vi "Dashboard Main.vi"() -> ()   [LabVIEW 2017]
uses:
  <vilib>/Utility/miscctls.llb/LVRowAndColumnTypeDef.ctl
  <vilib>/event_ctls.llb/eventvkey.ctl
  <vilib>/Rock Robotics/Network Tables/NT Read Numeric Array.vi
  <vilib>/Rock Robotics/WPI/Dashboard/WPI_DashboardLogging Global.vi
panel:
  in  "Camera Settings Right":T1={"Frame Rate"=30, "Compression"=30, "Size"=1, "DB Camera Config"=FALSE} {"Frame Rate" scale=1.0..30.0; "Compression" scale=100.0..-1.0; "Size" items=["640x480", "320x240", "160x120"]}
  in  "Camera Name Right":string(combo)="No Camera Selection"
  out "Camera Info":cluster{"Mbps LED":bool, "Mbps":dbl, "fps":dbl} {"fps" format="%#.1g"; "Mbps" format="%#.1g"}
  in  "Camera Settings":T1={"Frame Rate"=30, "Compression"=30, "Size"=1, "DB Camera Config"=FALSE} {"Frame Rate" scale=1.0..30.0; "Compression" scale=100.0..-1.0; "Size" items=["640x480", "320x240", "160x120"]}
  in  "TCP":refnum<k5>
  in  "Rec Mode":enum32{"Stop", "Record", "Playback"}(radio)
  out "Robot IP":string
  out "Image Message":string="Timeout in Camera Communications"
  in  "Dashboard Tab":T2(tab)
  out "NT Connection":bool
  out "MotorChart R":cluster{"Numeric":dbl, "Numeric":dbl}(graph)
  out "MotorChart L":cluster{"Numeric":dbl, "Numeric":dbl}(graph)
  out "MotorSliders R":cluster{"MotorSlide1":dbl, "MotorSlide2":dbl} {"MotorSlide2" scale=-1.0..1.0 scale format="%#_2e"; "MotorSlide1" scale=-1.0..1.0 scale format="%#_2e"}
  out "MotorSliders L":cluster{"MotorSlide1":dbl, "MotorSlide2":dbl} {"MotorSlide2" scale=-1.0..1.0 scale format="%#_2e"; "MotorSlide1" scale=-1.0..1.0 scale format="%#_2e"}
  out "Gyro":dbl(knob) scale=0.0..360.0
  out "JS1 Z":dbl(slide) scale=-1.0..1.0 scale format="%#_2e"
  out "JS1 Graph":cluster{"X":dbl, "Y":dbl}[](graph)
  out "JS1 Buttons":T3
  out "JS2 Z":dbl(slide) scale=-1.0..1.0 scale format="%#_2e"
  out "JS2 Graph":cluster{"X":dbl, "Y":dbl}[](graph)
  out "JS2 Buttons":T3
  out "Mode":T4(ring)=enum."Auto Disabled"
  out "Camera Image Right":T5(plugin-control)
  in  "DB/String 9":string
  in  "DB/String 8":string
  in  "DB/String 7":string
  in  "DB/String 6":string
  in  "DB/String 5":string
  in  "DB/String 4":string
  in  "DB/String 3":string
  in  "DB/String 2":string
  in  "DB/String 1":string
  in  "DB/String 0":string
  in  "DB/Slider 0":dbl(slide) scale=0.0..5.0
  in  "DB/Slider 1":dbl(slide) scale=0.0..5.0
  in  "DB/Slider 2":dbl(slide) scale=0.0..5.0
  in  "DB/Slider 3":dbl(slide) scale=0.0..5.0
  out "DB/LED 3":bool
  out "DB/LED 2":bool
  out "DB/LED 1":bool
  out "DB/LED 0":bool
  in  "DB/Button 3":bool
  in  "DB/Button 2":bool
  in  "DB/Button 1":bool
  in  "DB/Button 0":bool caption="New Name"
  in  "Test Slider":dbl(slide) scale=0.0..100.0 scale format="%#_3g"
  in  "On/Off":bool caption="Solenoid"
  in  "Test Name":u16(ring) items=["Select the test to run..."]
  in  "Test Tree":string(tree)
  in  "Motor":cluster{"Value":dbl, "Enable":bool} {"Value" scale=-1.0..1.0 scale format="%#_3g"}
  out "Progress":T6 {"Test Progress" scale=0.0..100.0}
  in  "Rev/Fwd":cluster{"Forward":bool, "Reverse":bool}
  in  "Test Ring":u16(ring) items=["Monochrome", "Color"]
  out "Cmd Status":string
  in  "Execute Command":bool
  in  "Command Params":string[][](table)
  in  "Command Selection":i32(listbox)
  in  "CheckList":i32(listbox)
  out "Tree":string(tree)
  out "Camera Image":T5(plugin-control)
  out "Background":bool
  in  "Camera Name":string(combo)="No Camera Selection"
  # "HW"
  # "HW"
  # "Joysticks"
  # "Drive Motors"
  # "Front"
  # "Right"
  # "Left"
  # "Back"
  # "Switch"
  # "Scale"
  # "This tab is a great place for autonomous settings and robot-specific values.\nPlace controls and indicators inside this tab and match name to\nDashboard Variables on robot. You can also delete this comment."
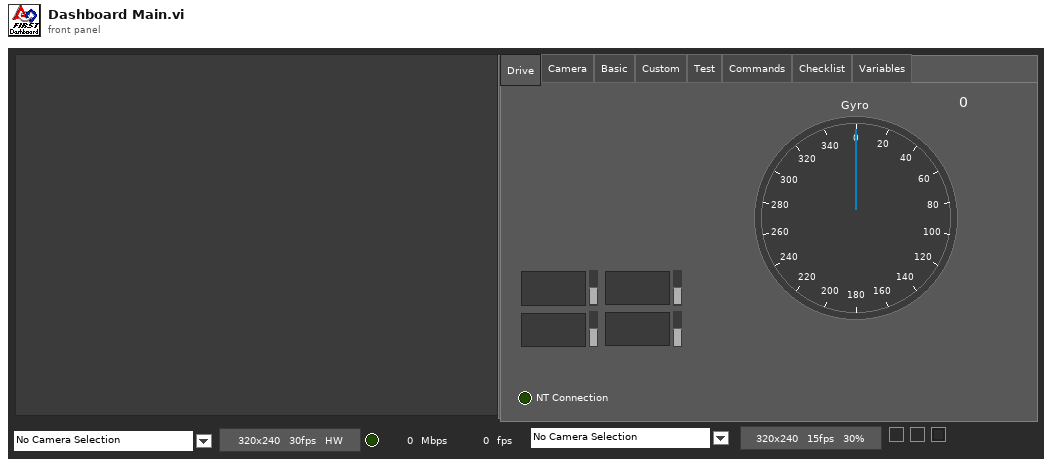
[diagram p1: front panel]
types:
  T1 = cluster{"Frame Rate":i32, "Compression":i32, "Size":u16, "DB Camera Config":bool}
  T2 = enum32{"Drive", "Camera", "Basic", "Custom", "Test", "Commands", "Checklist", "Variables"}
  T3 = cluster{bool, bool, bool, bool, bool, bool, bool, bool, bool, bool, bool, bool}
  T4 = enum8{"Tele-Op Disabled", "Tele-Op Enabled", "Auto Disabled", "Auto Enabled", "Test Disabled", "Test Enabled", "Disconnected", "No Code", "E-Stop"}
  T5 = typedef "IMAQ Image.ctl" = refnum<image>
  T6 = cluster{"Test Progress":u8, "Test Progress Text":string}
  T7 = cluster{"Save Path":path, "Interval (s)":dbl, "Keep":i32}
  T8 = typedef "Image Type" = u32
  T9 = cluster{"IDs":cluster{"RPC field ID":u16, "Unique ID":u16}, "String":string}
  T10 = cluster{"Error Strings":string, "Disable Counts":cluster{u16, u16}, "Rail Faults":cluster{u16, u16, u16}, "Robot IP":string, "DB Mode":u8, "Event Info":cluster{"Name":string, "Type":u8, "Number":u16, "Replay":u8}}
  T11 = cluster{"Storage":cluster{"Disk Free":u64, "RAM Block":u32, "RAM free":u32}, "CPU Utilization":cluster{"CPU % ISR":sgl, "CPU % Time Crit":sgl, "CPU % Timed Str":sgl, "CPU % High":sgl, "CPU % Above":sgl, "CPU % Normal":sgl, "CPU % Low":sgl}, "CAN":cluster{"% Bus Utilization":sgl, "Bus Off Cnt":u32, "TX_FIFO Full Cnt":u32, "Receive Error Cnt":u8, "Transmit Error Cnt":u8}, "HID":cluster{"HID Outputs":u32, "Rumble Low":u16, "Rumble High":u16}[]}
  T12 = cluster{"Status bits":cluster{"Test Mode":bool, "Autonomous":bool, "Enabled":bool, "Code Start":bool, "Brownout":bool, "Reserved 2":bool, "Reserved 3":bool, "E-Stop":bool}, "Code Trace":cluster{"Disabled":bool, "TeleOp":bool, "Auto":bool, "Test":bool}, "Controller Type":enum16{"unknown", "cRIO", "roboRio"}, "Code?":enum16{"unknown", "noCode", "code"}, "Battery V":dbl}
  T13 = cluster{"Control Bits":cluster{"TestMode":bool, "Autonomous":bool, "Enabled":bool, "FMS Present":bool, bool, bool, bool, "E-Stop":bool}, "Team Station ":u8, "Countdown":sgl, "Joystick Values":cluster{"Axes":dbl[], "Buttons":bool[], "POVs":i16[]}[]}
  T14 = cluster{"Axes":dbl[], "Buttons":bool[], "POVs":i16[]}[]
  T15 = cluster{"Axes":dbl[], "Buttons":bool[], "POVs":i16[]}
  T16 = cluster{"Buttons[0]":bool, "Buttons[1]":bool, "Buttons[2]":bool, "Buttons[3]":bool, "Buttons[4]":bool, "Buttons[5]":bool, "Buttons[6]":bool, "Buttons[7]":bool, "Buttons[8]":bool, "Buttons[9]":bool, "Buttons[10]":bool, "Buttons[11]":bool}
  T17 = cluster{"Camera Image":refnum<vi>, "Dashboard Tab":refnum<vi>, "Background":refnum<vi>, "Rec Mode":refnum<vi>, "Test Slider":refnum<vi>, "On/Off ":refnum<vi>, "Test Ring":refnum<vi>, "Rev/Fwd":refnum<vi>, "Test Name":refnum<vi>, "Motor":refnum<vi>, "Progress":refnum<vi>, "CheckList":refnum<vi>, "Tree":refnum<vi>, "Test Tree":refnum<vi>, "Command Params":refnum<vi>, "Command Selection":refnum<vi>, "Execute Command":refnum<vi>, "Cmd Status":refnum<vi>, "Camera Settings":refnum<vi>, "Camera Name":refnum<vi>, "Camera Info":refnum<vi>, "Camera Settings Right":refnum<vi>, "Camera Name Right":refnum<vi>, "Camera Image Right":refnum<vi>}
  T18 = cluster{"Camera Name":string, string, "Saved DB Images Info":cluster{"Save Path":path, "Interval (s)":dbl, "Keep":i32}}
  T19 = cluster{"Camera Name Right":string, string, "Saved DB Images Info":cluster{"Save Path":path, "Interval (s)":dbl, "Keep":i32}}
  T20 = cluster{"Operation":enum16{"Update", "Clear"}, "Color Box":u32}[]
  T21 = typedef "eventvkey.ctl" = enum16{"ASCII", "Enter", "Return", "Shift", "Ctrl", "Alt", "Cmd", "Opt", "Caps", "NumLock", "Clear", "Break", "Up", "Down", "Left", "Right", "Insert", "Delete", "Home", "End", "PageUp", "PageDown", "Escape", "Help", "Pause", "ScrollLock", "F1", "F2", "F3", "F4", "F5", "F6", "F7", "F8", "F9", "F10", "F11", "F12", "F13", "F14", "F15", "F16", "F17", "F18", "F19", "F20", "F21", "F22", "F23", "F24", "Play", "VolumeUp", "VolumeDown", "Mute", "Two Byte Char"}
  T22 = cluster{"Image Size":bool, "Image Type":bool, "Pixel Value":bool, "ROI Information":bool, "Zoom Factor":bool}
  T23 = cluster{"Operation":enum16{"Update", "Clear"}, "Color Box":u32}
  T24 = typedef "LVRowAndColumnTypeDef.ctl" = cluster{"Row":i32, "Column":i32}
  T25 = cluster{"Shift":bool, "Ctrl":bool, "Alt":bool, "Cmd":bool, "Opt":bool}
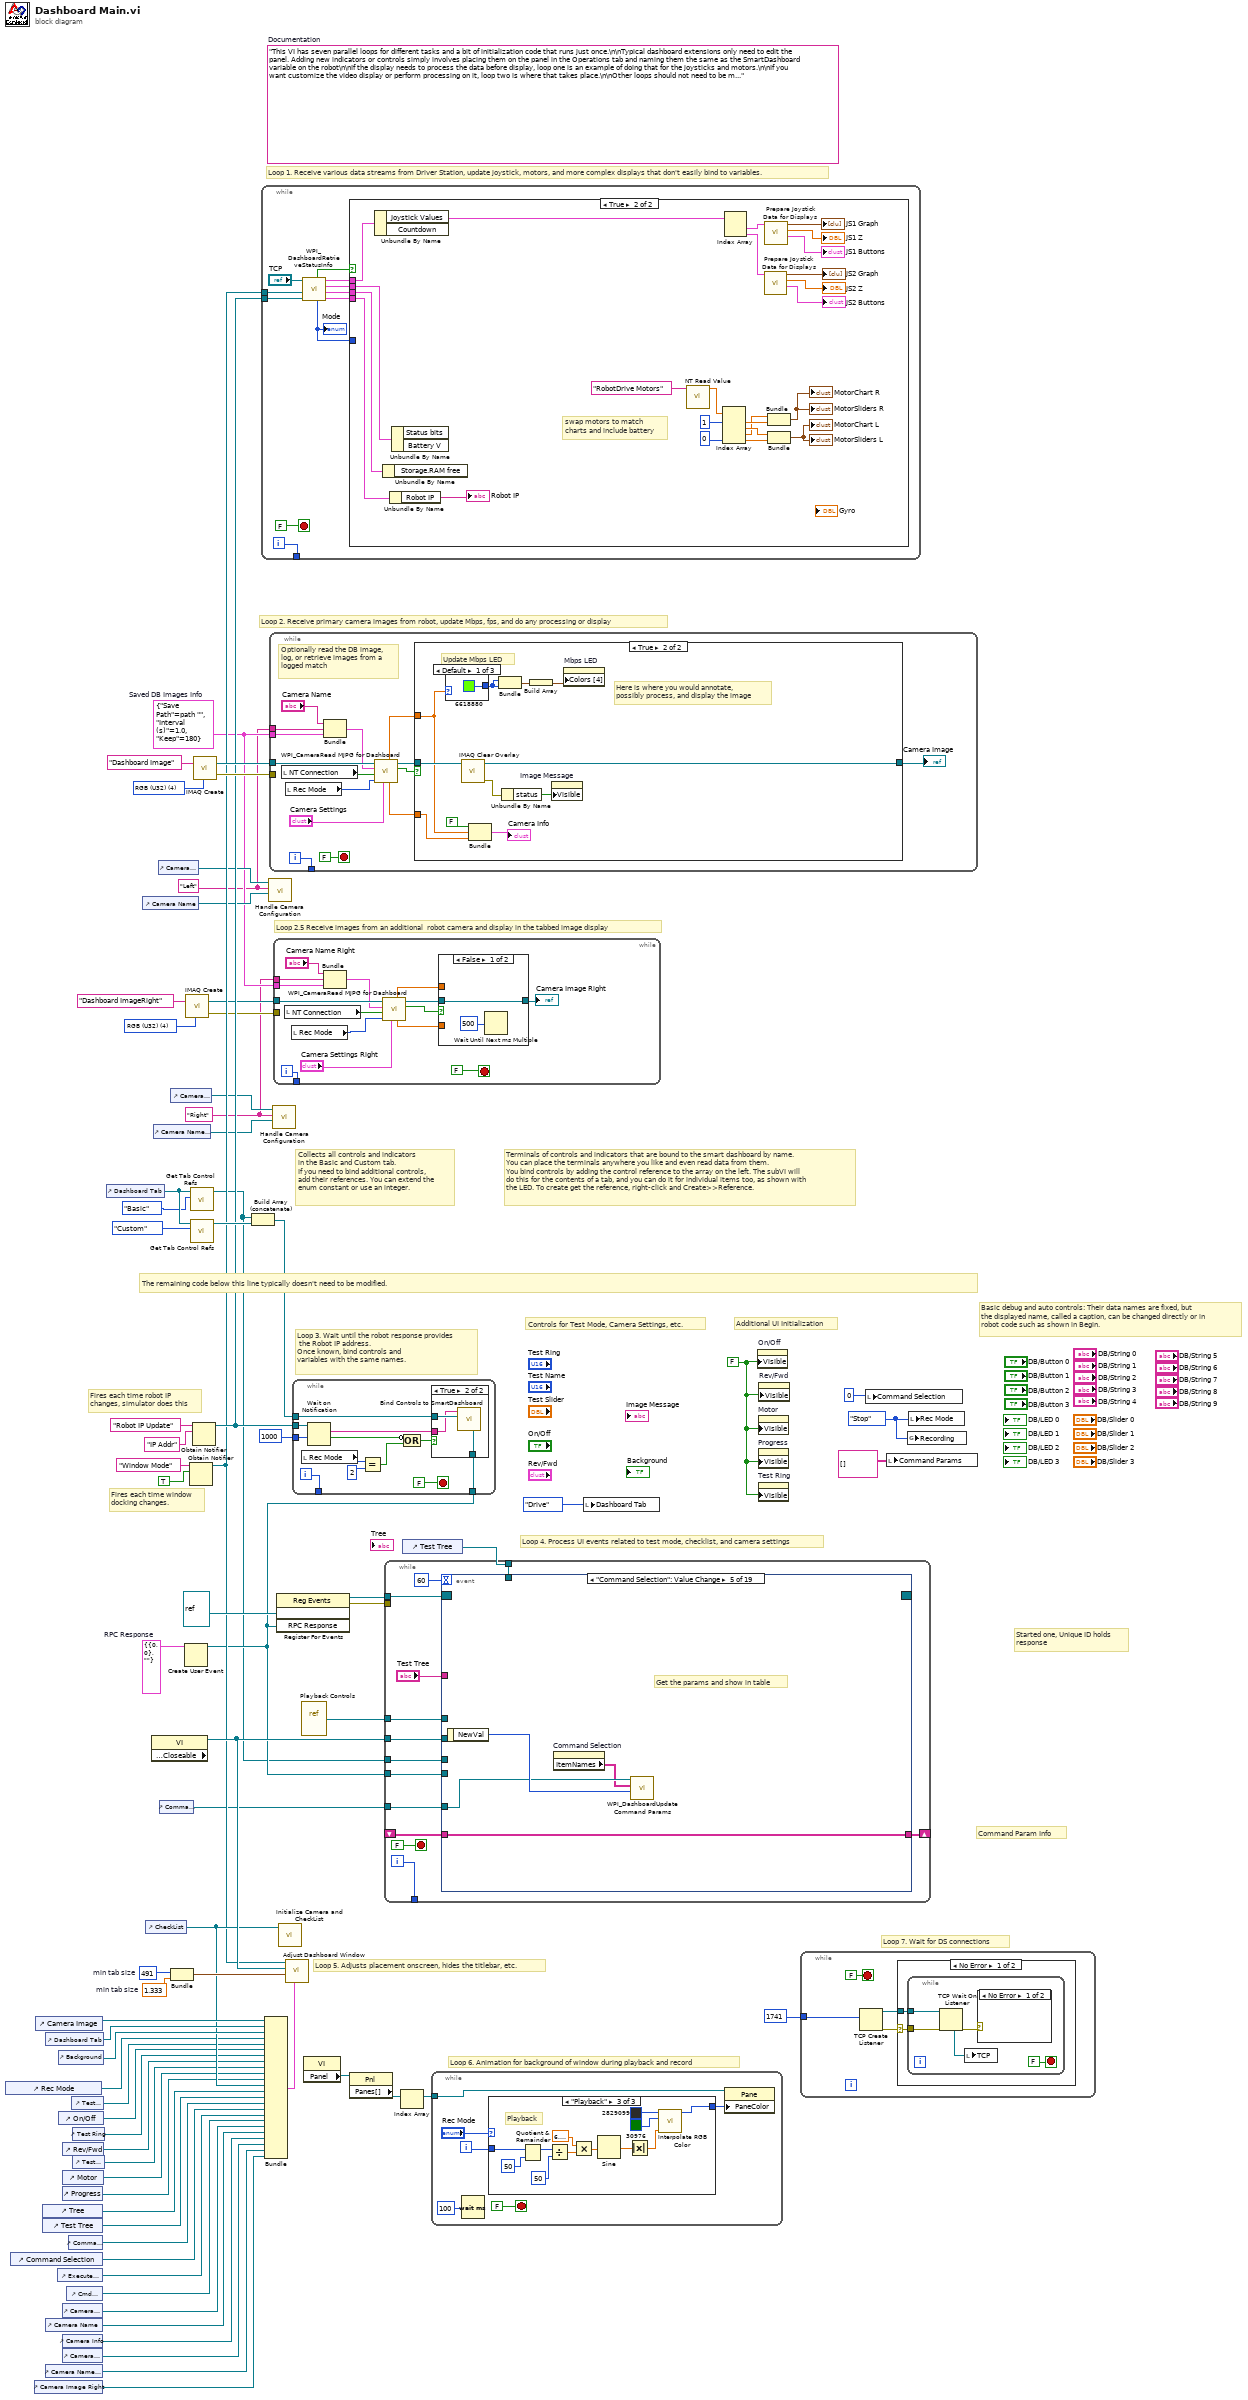
[diagram p0: block diagram]
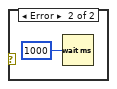
[diagram p3: hidden frame]
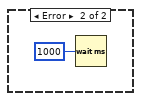
[diagram p4: hidden frame]
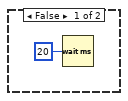
[diagram p5: hidden frame]
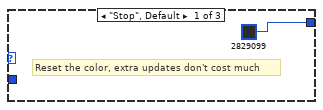
[diagram p6: hidden frame]
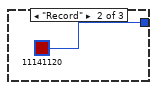
[diagram p7: hidden frame]
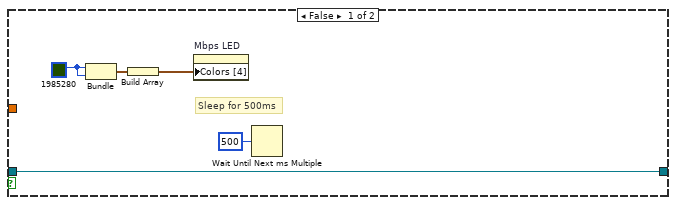
[diagram p9: hidden frame]
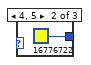
[diagram p10: hidden frame]
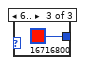
[diagram p11: hidden frame]
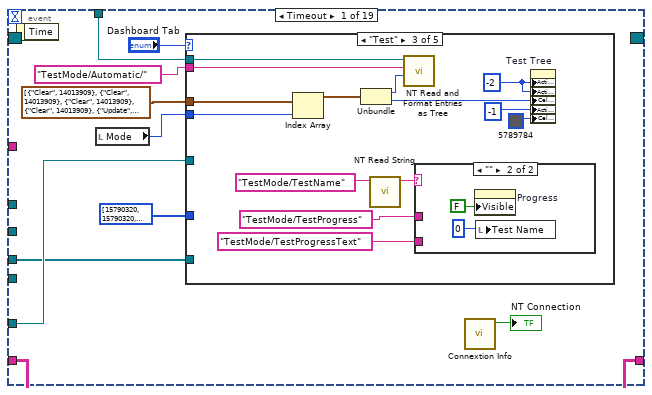
[diagram p12: hidden frame]
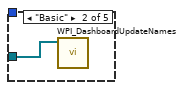
[diagram p14: hidden frame]
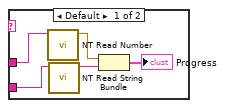
[diagram p15: hidden frame]
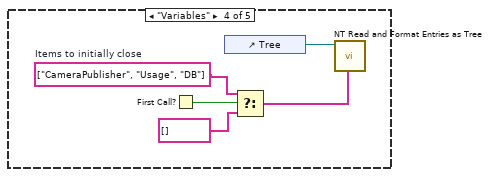
[diagram p16: hidden frame]
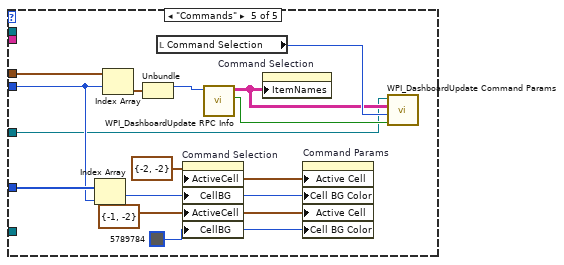
[diagram p17: hidden frame]
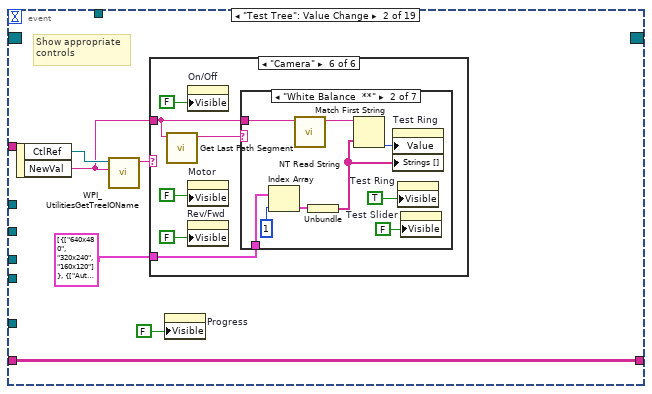
[diagram p18: hidden frame]
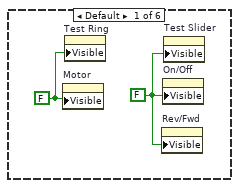
[diagram p19: hidden frame]
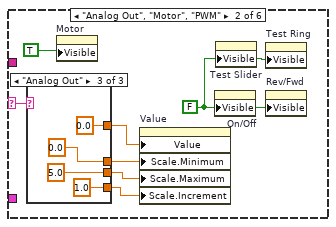
[diagram p20: hidden frame]
diagram:
  w3 = T7 {"Save Path"=path "", "Interval (s)"=1.0, "Keep"=180}  # Saved DB Images Info
  w2 = "Right"
  w1 = "Left"
  w13 = T8 4 items=["Grayscale (U8)", "Grayscale (I16)", "Grayscale (SGL)", "Complex (CSG)", "RGB (U32)", "HSL (U32)", "RGB (U64)"] ("Image Type")
  w27 = T9 {"IDs"={"RPC field ID"=0, "Unique ID"=0}, "String"=""}  # RPC Response
  w50 = 491  # min tab size
  w49 = 1.333  # min tab size
  w57 = enum32{"Stop", "Record", "Playback"}."Stop" ("Rec Mode")
  w34 = FALSE ("Visible")
  (unwired) "This VI has seven parallel loops for different tasks and a bit of initialization code that runs just once.\n\nTypical dashboard extensions only need to edit the panel. Adding new indicators or controls simply involves placing them on the panel in the Operations tab and naming them the same as the SmartDashboard variable on the robot\n\nIf the display needs to process the data before display, loop one is an example of doing that for the joysticks and motors.\n\nIf you want customize the video display or perform processing on it, loop two is where that takes place.\n\nOther loops should not need to be modified. They are pretty standard, and document the task they perform."  # Documentation
  w74 = T8 4 items=["Grayscale (U8)", "Grayscale (I16)", "Grayscale (SGL)", "Complex (CSG)", "RGB (U32)", "HSL (U32)", "RGB (U64)"] ("Image Type")
  # "Loop 2.5 Receive images from an additional  robot camera and display in the tabbed image display"
  # "Command Param Info"
  # "Started one, Unique ID holds\nresponse"
  # "Loop 7. Wait for DS connections"
  # "Basic debug and auto controls: Their data names are fixed, but\nthe displayed name, called a caption, can be changed directly or in\nrobot code such as shown in Begin."
  # "Controls for Test Mode, Camera Settings, etc."
  # "Additional UI Initialization"
  # "Loop 6. Animation for background of window during playback and record"
  # "Fires each time robot IP\nchanges, simulator does this"
  # "Fires each time window\ndocking changes."
  # "Collects all controls and indicators\nin the Basic and Custom tab.\nIf you need to bind additional controls,\nadd their references. You can extend the\nenum constant or use an integer."
  # "The remaining code below this line typically doesn't need to be modified."
  # "Loop 4. Process UI events related to test mode, checklist, and camera settings"
  # "Terminals of controls and indicators that are bound to the smart dashboard by name.\nYou can place the terminals anywhere you like and even read data from them.\nYou bind controls by adding the control reference to the array on the left. The subVI will\ndo this for the contents of a tab, and you can do it for individual items too, as shown with\nthe LED. To create get the reference, right-click and Create>>Reference."
  # "Loop 3. Wait until the robot response provides\n the Robot IP address.\nOnce known, bind controls and\nvariables with the same names."
  # "Loop 5. Adjusts placement onscreen, hides the titlebar, etc."
  # "Loop 1. Receive various data streams from Driver Station, update joystick, motors, and more complex displays that don't easily bind to variables."
  # "Loop 2. Receive primary camera images from robot, update Mbps, fps, and do any processing or display"
  n1 = control-ref of="Rec Mode"() -> (w40:refnum<vi>)
  n2 = control-ref of="Command Selection"() -> (w26:refnum<vi>)
  n3 = control-ref of="Camera Image Right"() -> (w6:refnum<vi>)
  n4 = control-ref of="Camera Image"() -> (w52:refnum<vi>)
  n5 = control-ref of="Tree"() -> (w44:refnum<vi>)
  n6 = control-ref of="Test Tree"() -> (w43:refnum<vi>)
  n7 = control-ref of="Dashboard Tab"() -> (w51:refnum<vi>)
  n8 = control-ref of="Camera Name"() -> (w17:refnum<vi>)
  n9 = control-ref of="Camera Name Right"() -> (w7:refnum<vi>)
  n10 = control-ref of="Execute Command"() -> (w28:refnum<vi>)
  n11 = control-ref of="Background"() -> (w47:refnum<vi>)
  n12 = control-ref of="On/Off"() -> (w38:refnum<vi>)
  n13 = control-ref of="Progress"() -> (w35:refnum<vi>)
  n14 = control-ref of="Camera Settings"() -> (w18:refnum<vi>)
  n15 = control-ref of="Camera Info"() -> (w16:refnum<vi>)
  n16 = control-ref of="Camera Settings Right"() -> (w8:refnum<vi>)
  n17 = control-ref of="Rev/Fwd"() -> (w36:refnum<vi>)
  n18 = control-ref of="Motor"() -> (w41:refnum<vi>)
  n19 = control-ref of="Cmd Status"() -> (w22:refnum<vi>)
  n20 = control-ref of="Command Params"() -> (w29:refnum<vi>)
  n21 = control-ref of="Test Slider"() -> (w39:refnum<vi>)
  n22 = control-ref of="Test Ring"() -> (w37:refnum<vi>)
  n23 = control-ref of="Test Name"() -> (w42:refnum<vi>)
  n24 = control-ref of="Dashboard Tab"() -> (w55:refnum<vi>)
  n25 = control-ref of="Camera Name"() -> (w19:refnum<vi>)
  n26 = control-ref of="CheckList"() -> (w45:refnum<vi>)
  n27 = property class="VI" props=["Front Panel.Closeable"]() -> (reference out=w56:refnum<vi>)  [unwired: 2 in, 2 out]
  n28 = control-ref of="Camera Name Right"() -> (w9:refnum<vi>)
  n29 = control-ref of="Camera Settings"() -> (w20:refnum<vi>)
  n30 = control-ref of="Command Params"() -> (w21:refnum<vi>)
  n31 = control-ref of="Camera Settings Right"() -> (w10:refnum<vi>)
  n32 = Bundle("min tab size"=w50, "min tab size"=w49) -> (w48:cluster{"min tab size":i32, "min tab size":dbl})  [unwired: 1 in]
  n33 = Create User Event(user event datatype=w27) -> (user event=w23:refnum<user-event>)  [unwired: 1 in, 1 out]
  n34 = call "IMAQ Create"("Image Name"="Dashboard ImageRight", "Image Type"=w13) -> ("New Image"=w12:T5, "error out"=w11:errorcluster)  [unwired: 2 in, 1 out]
  n35 = Obtain Notifier(name (unnamed)="Window Mode", notification data type=TRUE) -> (notifier out=w32:refnum<notifier>)  [unwired: 2 in, 2 out]
  n36 = call <vilib>:"Get Tab Control Refs.vi"("Page Index"=T2."Basic" ("Dashboard Tab"), "TabControl in"=w55) -> ("ControlsOnPage"=w15:refnum<vi>[])  [unwired: 9 in]
  n37 = call <vilib>:"Get Tab Control Refs.vi"("Page Index"=T2."Custom" ("Dashboard Tab"), "TabControl in"=w55) -> ("ControlsOnPage"=w54:refnum<vi>[])  [unwired: 9 in]
  n38 = Obtain Notifier(name (unnamed)="Robot IP Update", notification data type="IP Addr" ("name (unnamed)")) -> (notifier out=w33:refnum<notifier>)  [unwired: 2 in, 2 out]
  n39 = call "IMAQ Create"("Image Name"="Dashboard Image", "Image Type"=w74) -> ("New Image"=w72:T5, "error out"=w71:errorcluster)  [unwired: 2 in, 1 out]
  n40 = Build Array (concatenate)(w15, w54) -> (w53:refnum<vi>[])
  n41 = while {
    tunnel: [w84] -> _
    tunnel: w33 -> [w78]
    tunnel: w32 -> [w75]
    i -> [w84]
    stop <- FALSE stop-if-true
    n42 = call <vilib>:"WPI_DashboardRetrieveStatusInfo.vi"("Binding Refnum"=w78, "Window Mode Notifier"=w75, "TCP Cnx"="TCP") -> ("Power and Errors"=w79:T10, "Robot Metrics"=w82:T11, "Status Info"=w83:T12, "Control Info"=w80:T13, "Robot Mode"=w77:T4, "Process?"=w81:bool)  [unwired: 3 in]
    "Mode" <- w77
    n43 = case shown="True" w81 {
      tunnel: w83 -> [_ w110]
      tunnel: w82 -> [_ w109]
      tunnel: w80 -> [_ w108]
      tunnel: w79 -> [_ w107]
      tunnel: w77 -> [_ _]
      frame False {
        n44 = Wait (ms)(milliseconds to wait=u32 20) -> ()  [unwired: 1 out]
      }
      frame True {
        # "swap motors to match\ncharts and include battery"
        n45 = Unbundle By Name(w108) -> ("Joystick Values"=w98:T14)  [unwired: 1 out]
        n46 = Unbundle By Name(w109) -> ()  [unwired: 1 out]
        n47 = Unbundle By Name(w107) -> ("Robot IP"=→"Robot IP":string)
        n48 = Unbundle By Name(w110) -> ()  [unwired: 2 out]
        n49 = call-poly <vilib>:"NT Read Value.vi"("Name"="RobotDrive Motors") -> ("Numeric Array"=w88:dbl[])  [unwired: 9 in, 1 out]
        n50 = Index Array(array=w88, index #1=1, index #4=0) -> (element #1=w102:dbl, element #2=w103:dbl, element #3=w101:dbl, element #4=w106:dbl)  [unwired: 2 in]
        n51 = Index Array(array=w98) -> (element #1=w97:T15, element #2=w93:T15)  [unwired: 2 in]
        n52 = call "Prepare Joystick Data for Displays.vi"("Joystick Values"=w93) -> ("Buttons"=→"JS2 Buttons":T16, "Z Axis"=→"JS2 Z":dbl, "Cartesian Data"=→"JS2 Graph":cluster{"X axis":dbl, "X axis":dbl}[])  [unwired: 8 in]
        n53 = call "Prepare Joystick Data for Displays.vi"("Joystick Values"=w97) -> ("Buttons"=→"JS1 Buttons":T16, "Z Axis"=→"JS1 Z":dbl, "Cartesian Data"=→"JS1 Graph":cluster{"X axis":dbl, "X axis":dbl}[])  [unwired: 8 in]
        n54 = Bundle("Numeric"=w101, "Numeric"=w102) -> (→"MotorChart R" →"MotorSliders R":cluster{"Numeric":dbl, "Numeric":dbl})  [unwired: 1 in]
        n55 = Bundle("Numeric"=w103, "Numeric"=w106) -> (→"MotorChart L" →"MotorSliders L":cluster{"Numeric":dbl, "Numeric":dbl})  [unwired: 1 in]
      }
    }
  }
  n56 = Bundle("Camera Image"=w52, "Dashboard Tab"=w51, "Background"=w47, "Rec Mode"=w40, "Test Slider"=w39, "On/Off"=w38, "Test Ring"=w37, "Rev/Fwd"=w36, "Test Name"=w42, "Motor"=w41, "Progress"=w35, "CheckList"=w45, "Tree"=w44, "Test Tree"=w43, "Command Params"=w29, "Command Selection"=w26, "Execute Command"=w28, "Cmd Status"=w22, "Camera Settings"=w18, "Camera Name"=w17, "Camera Info"=w16, "Camera Settings Right"=w8, "Camera Name Right"=w7, "Camera Image Right"=w6) -> (w46:T17)  [unwired: 1 in]
  n57 = call "Handle Camera Configuration.vi"("CameraNameRef"=w19, "Display Name"=w1, "ClusterRef"=w20) -> ()  [unwired: 9 in]
  n58 = while {
    tunnel: w72 -> [w123]
    tunnel: w71 -> [_]
    tunnel: [w124] -> _
    tunnel: w3 -> [w114]
    tunnel: w1 -> [w111]
    i -> [w124]
    stop <- FALSE stop-if-true
    # "Optionally read the DB image,\nlog, or retrieve images from a\nlogged match"
    n59 = local read "NT Connection"() -> (w115:bool)
    n60 = local read "Rec Mode"() -> (w119:enum32{"Stop", "Record", "Playback"})
    n61 = Bundle("Camera Name"="Camera Name", w111, "Saved DB Images Info"=w114) -> (w113:T18)  [unwired: 1 in]
    n62 = call <vilib>:"WPI_CameraRead MJPG for Dashboard.vi"("Camera Settings"="Camera Settings", "Rec Mode"=w119, "NT Connection"=w115, "Capture Info"=w113, "Refnum in"=w123) -> ("Active"=w121:bool, "Refnum out"=w122:T5, "FPS"=w120:dbl, "Bandwidth (Mbps)"=w118:dbl)  [unwired: 3 in]
    n63 = case shown="True" w121 {
      tunnel: w122 -> [w126 w137]
      tunnel: w118 -> [_ w134]
      tunnel: w120 -> [_ w135]
      tunnel: [w126 w131] -> w116
      frame False {
        w128 = u32 1985280 ("Color Box")
        # "Sleep for 500ms"
        n64 = Bundle("Color Box"=w128, "Color Box"=w128) -> (w129:cluster{"Color Box":u32, "Color Box":u32})  [unwired: 1 out]
        n65 = Build Array(w129) -> (w127:cluster{"Color Box":u32, "Color Box":u32}[])
        n66 = property on="Mbps LED" class="Bool (strict)"("Colors [4]"=w127) -> ()  [unwired: 2 in, 2 out]
        n67 = Wait Until Next ms Multiple(millisecond multiple=u32 500) -> ()  [unwired: 1 out]
      }
      frame True {
        # "Here is where you would annotate,\npossibly process, and display the image"
        # "Update Mbps LED"
        n68 = case shown="Default" w134 {
          tunnel: [u32 6618880 ("Color Box") u32 16776722 ("Color Box") u32 16716800 ("Color Box")] -> w138
          frame Default {
          }
          frame 4, 5 {
          }
          frame 6.. {
          }
        }
        n69 = call "IMAQ Clear Overlay"("Image"=w137) -> ("error out"=w140:errorcluster, "Image Out"=w131:T5)  [unwired: 2 in, 7 out]
        n70 = Bundle(FALSE, "Bandwidth (Mbps)"=w134, "FPS"=w135) -> (→"Camera Info":cluster{bool, "Bandwidth (Mbps)":dbl, "FPS":dbl})  [unwired: 1 in]
        n71 = Bundle("Color Box"=w138, "Color Box"=w138) -> (w139:cluster{"Color Box":u32, "Color Box":u32})  [unwired: 1 out]
        n72 = Unbundle By Name(w140) -> ("status"=w141:bool)
        n73 = Build Array(w139) -> (w136:cluster{"Color Box":u32, "Color Box":u32}[])
        n74 = property on="Image Message" class="Str"("Visible"=w141) -> ()  [unwired: 2 in, 2 out]
        n75 = property on="Mbps LED" class="Bool (strict)"("Colors [4]"=w136) -> ()  [unwired: 2 in, 2 out]
      }
    }
    "Camera Image" <- w116
  }
  n76 = call "Handle Camera Configuration.vi"("CameraNameRef"=w9, "Display Name"=w2, "ClusterRef"=w10) -> ()  [unwired: 9 in]
  n77 = while {
    tunnel: w12 -> [w159]
    tunnel: w11 -> [_]
    tunnel: [w154] -> _
    tunnel: w3 -> [w148]
    tunnel: w2 -> [w145]
    i -> [w154]
    stop <- FALSE stop-if-true
    n78 = local read "NT Connection"() -> (w149:bool)
    n79 = local read "Rec Mode"() -> (w158:enum32{"Stop", "Record", "Playback"})
    n80 = Bundle("Camera Name Right"="Camera Name Right", w145, "Saved DB Images Info"=w148) -> (w147:T19)  [unwired: 1 in]
    n81 = call <vilib>:"WPI_CameraRead MJPG for Dashboard.vi"("Camera Settings"="Camera Settings Right", "Rec Mode"=w158, "NT Connection"=w149, "Capture Info"=w147, "Refnum in"=w159) -> ("Active"=w153:bool, "Refnum out"=w156:T5, "FPS"=w151:dbl, "Bandwidth (Mbps)"=w152:dbl)  [unwired: 3 in]
    n82 = case shown="False" w153 {
      tunnel: w156 -> [w160 w162]
      tunnel: w152 -> [_ _]
      tunnel: w151 -> [_ _]
      tunnel: [w160 w162] -> w150
      frame False {
        n83 = Wait Until Next ms Multiple(millisecond multiple=u32 500) -> ()  [unwired: 1 out]
      }
      frame True {
      }
    }
    "Camera Image Right" <- w150
  }
  n84 = register-events(refnum<vi> refnum, w23) -> (reference out=w61:refnum<event-registration>, error out=w60:errorcluster)  [unwired: 2 in]
  n85 = call "Initialize Camera and CheckList.vi"("ListBox in"=w45) -> ()  [unwired: 11 in]
  n86 = call "Adjust Dashboard Window.vi"("Sizing Refnums"=w46, "Size Constraints"=w48, "VI"=w56, "WIn Mode"=w32) -> ()  [unwired: 8 in]
  n87 = while {
    tunnel: w53 -> [w174]
    tunnel: w33 -> [w172]
    tunnel: [w170] -> _
    tunnel: u32 1000 ("milliseconds to wait") -> [w169]
    tunnel: w23 -> [w163]
    i -> [w170]
    stop <- FALSE stop-if-true
    n88 = local read "Rec Mode"() -> (w165:enum32{"Stop", "Record", "Playback"})
    n89 = Wait on Notification(notifier=w172, timeout in ms (-1)=w169) -> (notification=w171:string, timed out?=w167:bool)  [unwired: 2 in, 2 out]
    n90 = Equal?(x=w165, y=u16 2 ("Rec Mode")) -> (x = y?=w166:bool)
    n91 = Compound Arithmetic op=OR(invert w167, w166) -> (w168:bool)
    n92 = case shown="True" w168 {
      tunnel: w174 -> [_ w177]
      tunnel: w171 -> [_ w176]
      tunnel: w163 -> [_ w175]
      frame False {
      }
      frame True {
        n93 = call <vilib>:"Bind Controls to SmartDashboard.vi"("RPC ref"=w175, "Bound Control Refs"=w177, "Server IP Address"=w176) -> ()  [unwired: 9 in]
      }
    }
  }
  n94 = vi-ref "Playback Controls.vi"() -> (w62:refnum<vi>)
  n95 = property class="VI"() -> ("Panel"=w64:refnum<vi>)  [unwired: 2 in, 2 out]
  n96 = property class="Pnl"(reference=w64) -> ("Panes[]"=w65:refnum<vi>[])  [unwired: 1 in, 2 out]
  n97 = Index Array(array=w65) -> (element=w63:refnum<vi>)  [unwired: 1 in]
  n98 = control-ref of="Test Tree"() -> (w66:refnum<vi>)
  n99 = while {
    tunnel: [w187] -> _
    tunnel: w66 -> [w186]
    tunnel: w62 -> [w185]
    tunnel: w61 -> [w184]
    tunnel: w60 -> [_]
    tunnel: w56 -> [w183]
    tunnel: w23 -> [w182]
    tunnel: w21 -> [w181]
    shift-right: [w180] -> _
    shift-left: _ -> [w179]
    tunnel: w15 -> [w178]
    i -> [w187]
    stop <- FALSE stop-if-true
    n100 = event shown="[4] \"Command Selection\": Value Change" {
      selector: w184 -> [_ _ _ _ _ _ _ _ _ _ _ _ _ _ _ _ _ _ _]
      dyn-events: [_ _ _ _ _ _ _ _ _ _ _ _ _ _ w441 _ _ _ _] -> _
      timeout: u32 60 ("milliseconds to wait") -> [_ _ _ _ _ _ _ _ _ _ _ _ _ _ _ _ _ _ _]
      tunnel: w186 -> [w199 _ _ _ _ _ _ _ _ _ _ _ _ _ _ _ _ _ _]
      tunnel: "Test Tree" -> [_ _ _ _ _ _ _ _ _ w408 w416 w418 w422 w430 _ _ _ _ _]
      tunnel: w185 -> [_ _ _ _ _ _ _ _ _ _ _ _ _ _ w443 _ w461 _ _]
      tunnel: w183 -> [_ _ _ _ _ _ _ _ _ _ _ _ _ _ w439 _ _ _ _]
      tunnel: w182 -> [_ _ _ _ _ _ _ _ _ _ _ _ _ _ w437 _ _ _ _]
      tunnel: w181 -> [w194 _ _ _ w359 _ _ _ _ _ _ _ _ _ _ _ _ _ _]
      tunnel: [w193 w242 w344 w349 w357 w366 w376 w383 w395 w407 w414 w417 w421 w429 w436 w456 w458 w462 w475] -> w180
      tunnel: w179 -> [w193 w242 w344 w349 w357 _ _ w383 w395 w407 w414 w417 w421 w429 w436 w456 w458 w462 w475]
      tunnel: w178 -> [w191 _ _ _ _ _ _ _ _ _ _ _ _ _ _ _ _ _ _]
      event Timeout {
        n101 = event-data() -> ()  [unwired: 1 in, 1 out]
        n102 = local read "Mode"() -> (w196:T4)
        n103 = case shown="\"Test\"" "Dashboard Tab" {
          tunnel: w199 -> [_ _ w215 _ _]
          tunnel: "TestMode/Automatic/" ("Name Pattern") -> [_ _ w214 _ _]
          tunnel: T20 [{"Operation"=enum."Clear", "Color Box"=14013909}, {"Operation"=enum."Clear", "Color Box"=14013909}, {"Operation"=enum."Clear", "Color Box"=14013909}, {"Operation"=enum."Clear", "Color Box"=14013909}, {"Operation"=enum."Update", "Color Box"=14013909}, {"Operation"=enum."Update", "Color Box"=16777215}, {"Operation"=enum."Clear", "Color Box"=14013909}, {"Operation"=enum."Clear", "Color Box"=14013909}, {"Operation"=enum."Clear", "Color Box"=14013909}] -> [_ _ w207 _ w235]
          tunnel: w196 -> [_ _ w206 _ w234]
          tunnel: u32[] [15790320, 15790320, 15790320, 15790320, 16777215, 16777215, 15790320, 15790320, 15790320] -> [_ _ _ _ w240]
          tunnel: w194 -> [_ _ _ _ w228]
          tunnel: w191 -> [_ w201 _ _ _]
          frame "Custom", Default {
          }
          frame "Basic" {
            n104 = call <vilib>:"WPI_DashboardUpdateNames.vi"("Controls on Tab"=w201) -> ()  [unwired: 11 in]
          }
          frame "Test" {
            w213 = -2 ("Active Item:Row Number")
            n105 = Index Array(array=w207, index=w206) -> (element=w208:T23)
            n106 = Unbundle(w208) -> ("Operation"=w209:enum16{"Update", "Clear"}, "Color Box"=w210:u32)
            n107 = call <vilib>:"NT Read String.vi"("Name"="TestMode/TestName") -> ("String"=w204:string)  [unwired: 9 in, 1 out]
            n108 = call <vilib>:"NT Read and Format Entries as Tree.vi"("Operation"=w209, "Name Pattern"=w214, "Tree Refnum"=w215) -> ()  [unwired: 7 in, 2 out]
            n109 = case shown="\"\"" w204 {
              tunnel: "TestMode/TestProgress" ("Name") -> [w217 _]
              tunnel: "TestMode/TestProgressText" ("Name") -> [w216 _]
              frame Default {
                n110 = call <vilib>:"NT Read Number.vi"("Name"=w217) -> ("Numeric"=w218:dbl)  [unwired: 9 in, 1 out]
                n111 = call <vilib>:"NT Read String.vi"("Name"=w216) -> ("String"=w219:string)  [unwired: 9 in, 1 out]
                n112 = Bundle("Numeric"=w218, "String"=w219) -> (→"Progress":cluster{"Numeric":dbl, "String":string})  [unwired: 1 in]
              }
              frame "" {
                n113 = property on="Progress" class="Clust (strict)"("Visible"=FALSE) -> ()  [unwired: 2 in, 2 out]
                n114 = local write "Test Name"(u16 0) -> ()
              }
            }
            n115 = property on="Test Tree" class="Tree (strict)"("Active Item Row Number"=w213, "ActiveColNum"=w213, "CellBG"=w210, "Active Item Row Number"=-1 ("Active Item:Row Number"), "CellBG"=u32 5789784 ("Color Box")) -> ()  [unwired: 2 in, 2 out]
          }
          frame "Variables" {
            w225 = string[] ["CameraPublisher", "Usage", "DB"]  # Items to initially close
            n116 = First Call?() -> (First Call?: T/F=w226:bool)
            n117 = control-ref of="Tree"() -> (w227:refnum<vi>)
            n118 = Select(t=w225, s=w226, f=string[] []) -> (s? t:f=w223:string[])
            n119 = call <vilib>:"NT Read and Format Entries as Tree.vi"("Tags to  Close"=w223, "Tree Refnum"=w227) -> ()  [unwired: 8 in, 2 out]
          }
          frame "Commands" {
            w236 = u32 5789784 ("Color Box")
            w237 = T24 {"Row"=-1, "Column"=-2} ("Active Cell:Active Cell")
            w239 = T24 {"Row"=-2, "Column"=-2} ("Active Cell:Active Cell")
            n120 = Index Array(array=w240, index=w234) -> (element=w238:u32)
            n121 = Index Array(array=w235, index=w234) -> (element=w233:T23)
            n122 = Unbundle(w233) -> ("Operation"=w232:enum16{"Update", "Clear"})  [unwired: 1 out]
            n123 = local read "Command Selection"() -> (w231:i32)
            n124 = property on="Command Selection" class="MCListbox (strict)"("ActiveCell"=w239, "CellBG"=w238, "ActiveCell"=w237, "CellBG"=w236) -> ()  [unwired: 2 in, 2 out]
            n125 = call <vilib>:"WPI_DashboardUpdate RPC Info.vi"("Operation"=w232) -> ("update"=w230:bool, "commands"=w229:string[][])  [unwired: 9 in]
            n126 = property on="Command Selection" class="MCListbox (strict)"("ItemNames"=w229) -> ()  [unwired: 2 in, 2 out]
            n127 = property on="Command Params" class="Tbl (strict)"("Active Cell"=w239, "Cell BG Color"=w238, "Active Cell"=w237, "Cell BG Color"=w236) -> ()  [unwired: 2 in, 2 out]
            n128 = call <vilib>:"WPI_DashboardUpdate Command Params.vi"("Update"=w230, "NewVal"=w231, "Commands"=w229, "Param Tbl"=w228) -> ()  [unwired: 7 in, 1 out]
          }
        }
        n129 = call <vilib>:"Connextion Info.vi"() -> ("Connected"=→"NT Connection":bool)  [unwired: 10 in, 1 out]
      }
      event "Test Tree": Value Change {
        # "Show appropriate\ncontrols"
        n130 = event-data() -> ("CtlRef"=w245:refnum<vi>, "NewVal"=w243:string)  [unwired: 1 in]
        n131 = call <vilib>:"WPI_UtilitiesGetTreeIOName.vi"("NewVal"=w243, "TreeControl in"=w245) -> ("I/O Name"=w246:string)  [unwired: 9 in]
        n132 = case shown="\"Camera\"" w246 {
          selector: w246 -> [_ w253 _ w275 w284 _]
          tunnel: w243 -> [_ _ w272 w274 _ w291]
          tunnel: cluster{string[]}[] [{["640x480", "320x240", "160x120"]}, {["Auto", "Fixed indoor", "Fixed outdoor 1", "Fixed outdoor 2", "Fixed fluorescent 1", "Fixed fluorescent 2", "Hold current"]}, {["Auto", "Flicker-free 50 Hz", "Flicker-free 60 Hz", "Hold current"]}, {["None", "Prioritize frame rate", "Prioritize image quality"]}, {["Monochrome", "Color"]}] -> [_ _ _ _ _ w290]
          frame Default {
            w248 = FALSE ("Visible")
            w247 = FALSE ("Visible")
            n133 = property on="Motor" class="Clust (strict)"("Visible"=w247) -> ()  [unwired: 2 in, 2 out]
            n134 = property on="Test Ring" class="Ring (strict)"("Visible"=w247) -> ()  [unwired: 2 in, 2 out]
            n135 = property on="Rev/Fwd" class="Clust (strict)"("Visible"=w248) -> ()  [unwired: 2 in, 2 out]
            n136 = property on="On/Off" class="Bool (strict)"("Visible"=w248) -> ()  [unwired: 2 in, 2 out]
            n137 = property on="Test Slider" class="Slide (strict)"("Visible"=w248) -> ()  [unwired: 2 in, 2 out]
          }
          frame "Analog Out", "Motor", "PWM" {
            w254 = FALSE ("Visible")
            n138 = case shown="\"Analog Out\"" w253 {
              tunnel: [1.0 ("Value") -1.0 ("Value") 0.0 ("Value")] -> w252
              tunnel: [255.0 ("Value") 1.0 ("Value") 5.0 ("Value")] -> w251
              tunnel: [128.0 ("Value") 0.0 ("Value") 0.0 ("Value")] -> w250
              tunnel: [64.0 ("Value") 0.5 ("Value") 1.0 ("Value")] -> w249
              frame "PWM" {
              }
              frame "Motor", Default {
              }
              frame "Analog Out" {
              }
            }
            n139 = property on="Motor" class="Clust (strict)"("Visible"=TRUE) -> ()  [unwired: 2 in, 2 out]
            n140 = property on="Value" class="Slide (strict)"("Value"=w250, "Scale.Minimum"=w252, "Scale.Maximum"=w251, "Scale.Increment"=w249) -> ()  [unwired: 2 in, 2 out]
            n141 = property on="On/Off" class="Bool (strict)"("Visible"=w254) -> ()  [unwired: 2 in, 2 out]
            n142 = property on="Test Slider" class="Slide (strict)"("Visible"=w254) -> ()  [unwired: 2 in, 2 out]
            n143 = property on="Test Ring" class="Ring (strict)"("Visible"=w254) -> ()  [unwired: 2 in, 2 out]
            n144 = property on="Rev/Fwd" class="Clust (strict)"("Visible"=w254) -> ()  [unwired: 2 in, 2 out]
          }
          frame "Servo" {
            w270 = FALSE ("Visible")
            n145 = call <vilib>:"NT Read Number.vi"("Name"=w272) -> ("Numeric"=w271:dbl)  [unwired: 9 in, 1 out]
            n146 = property on="Test Slider" class="Slide (strict)"("Visible"=TRUE, "Scale.Maximum"=170.0 ("Scale.Range:Maximum")) -> ()  [unwired: 2 in, 2 out]
            n147 = local write "Test Slider"(w271) -> ()
            n148 = property on="Motor" class="Clust (strict)"("Visible"=w270) -> ()  [unwired: 2 in, 2 out]
            n149 = property on="Rev/Fwd" class="Clust (strict)"("Visible"=w270) -> ()  [unwired: 2 in, 2 out]
            n150 = property on="On/Off" class="Bool (strict)"("Visible"=w270) -> ()  [unwired: 2 in, 2 out]
            n151 = property on="Test Ring" class="Ring (strict)"("Visible"=w270) -> ()  [unwired: 2 in, 2 out]
          }
          frame "Relay", "Solenoid" {
            w273 = FALSE ("Visible")
            n152 = property on="Motor" class="Clust (strict)"("Visible"=w273) -> ()  [unwired: 2 in, 2 out]
            n153 = property on="Test Slider" class="Slide (strict)"("Visible"=w273) -> ()  [unwired: 2 in, 2 out]
            n154 = Search and Replace String(input string=w274, search string="/Value  **", replace string="/Direction") -> (result string=w280:string)  [unwired: 5 in, 3 out]
            n155 = property on="Test Ring" class="Ring (strict)"("Visible"=w273) -> ()  [unwired: 2 in, 2 out]
            n156 = call <vilib>:"NT Read String.vi"("Name"=w280) -> ("String"=w278:string)  [unwired: 9 in, 1 out]
            n157 = Equal?(x="Both directions", y=w278) -> (x = y?=w276:bool)
            n158 = Not(x=w276) -> (.not. x?=w277:bool)
            n159 = property on="Rev/Fwd" class="Clust (strict)"("Visible"=w276) -> ()  [unwired: 2 in, 2 out]
            n160 = property on="On/Off" class="Bool (strict)"("Visible"=w277, "Caption.Text"=w275) -> ()  [unwired: 2 in, 2 out]
          }
          frame "Compressor", "Digital Out" {
            w283 = FALSE ("Visible")
            # "Get direction and finish"
            n161 = property on="Motor" class="Clust (strict)"("Visible"=w283) -> ()  [unwired: 2 in, 2 out]
            n162 = property on="Test Slider" class="Slide (strict)"("Visible"=w283) -> ()  [unwired: 2 in, 2 out]
            n163 = property on="Test Ring" class="Ring (strict)"("Visible"=w283) -> ()  [unwired: 2 in, 2 out]
            n164 = property on="On/Off" class="Bool (strict)"("Visible"=TRUE, "Caption.Text"=w284) -> ()  [unwired: 2 in, 2 out]
            n165 = property on="Rev/Fwd" class="Clust (strict)"("Visible"=FALSE) -> ()  [unwired: 2 in, 2 out]
          }
          frame "Camera" {
            n166 = call <vilib>:"Get Last Path Segment.vi"("String in"=w291) -> ("String out"=w292:string)  [unwired: 10 in]
            n167 = property on="On/Off" class="Bool (strict)"("Visible"=FALSE) -> ()  [unwired: 2 in, 2 out]
            n168 = property on="Motor" class="Clust (strict)"("Visible"=FALSE) -> ()  [unwired: 2 in, 2 out]
            n169 = property on="Rev/Fwd" class="Clust (strict)"("Visible"=FALSE) -> ()  [unwired: 2 in, 2 out]
            n170 = case shown="\"White Balance  **\"" w292 {
              tunnel: w291 -> [w298 w307 w316 w325 w334 _ w340]
              tunnel: w290 -> [w296 w304 w313 w322 w331 _ _]
              frame "Size  **" {
                n171 = Index Array(array=w296) -> (element=w295:cluster{string[]})  [unwired: 1 in]
                n172 = call <vilib>:"NT Read String.vi"("Name"=w298) -> ("String"=w297:string)  [unwired: 9 in, 1 out]
                n173 = Unbundle(w295) -> (w293:string[])
                n174 = Match First String(2:w293, 3:w297) -> (0:w294:i32)  [unwired: 1 out]
                n175 = property on="Test Ring" class="Ring (strict)"("Value"=w294, "Strings []"=w293) -> ()  [unwired: 2 in, 2 out]
                n176 = property on="Test Ring" class="Ring (strict)"("Visible"=TRUE) -> ()  [unwired: 2 in, 2 out]
                n177 = property on="Test Slider" class="Slide (strict)"("Visible"=FALSE) -> ()  [unwired: 2 in, 2 out]
              }
              frame "White Balance  **" {
                n178 = Index Array(array=w304, index=1) -> (element=w305:cluster{string[]})
                n179 = call <vilib>:"NT Read String.vi"("Name"=w307) -> ("String"=w306:string)  [unwired: 9 in, 1 out]
                n180 = Unbundle(w305) -> (w302:string[])
                n181 = Match First String(2:w302, 3:w306) -> (0:w301:i32)  [unwired: 1 out]
                n182 = property on="Test Ring" class="Ring (strict)"("Value"=w301, "Strings []"=w302) -> ()  [unwired: 2 in, 2 out]
                n183 = property on="Test Ring" class="Ring (strict)"("Visible"=TRUE) -> ()  [unwired: 2 in, 2 out]
                n184 = property on="Test Slider" class="Slide (strict)"("Visible"=FALSE) -> ()  [unwired: 2 in, 2 out]
              }
              frame "Exposure  **" {
                n185 = Index Array(array=w313, index=2) -> (element=w314:cluster{string[]})
                n186 = call <vilib>:"NT Read String.vi"("Name"=w316) -> ("String"=w315:string)  [unwired: 9 in, 1 out]
                n187 = Unbundle(w314) -> (w310:string[])
                n188 = Match First String(2:w310, 3:w315) -> (0:w311:i32)  [unwired: 1 out]
                n189 = property on="Test Ring" class="Ring (strict)"("Value"=w311, "Strings []"=w310) -> ()  [unwired: 2 in, 2 out]
                n190 = property on="Test Ring" class="Ring (strict)"("Visible"=TRUE) -> ()  [unwired: 2 in, 2 out]
                n191 = property on="Test Slider" class="Slide (strict)"("Visible"=FALSE) -> ()  [unwired: 2 in, 2 out]
              }
              frame "Exposure Priority  **" {
                n192 = Index Array(array=w322, index=3) -> (element=w323:cluster{string[]})
                n193 = call <vilib>:"NT Read String.vi"("Name"=w325) -> ("String"=w324:string)  [unwired: 9 in, 1 out]
                n194 = Unbundle(w323) -> (w319:string[])
                n195 = Match First String(2:w319, 3:w324) -> (0:w320:i32)  [unwired: 1 out]
                n196 = property on="Test Ring" class="Ring (strict)"("Value"=w320, "Strings []"=w319) -> ()  [unwired: 2 in, 2 out]
                n197 = property on="Test Ring" class="Ring (strict)"("Visible"=TRUE) -> ()  [unwired: 2 in, 2 out]
                n198 = property on="Test Slider" class="Slide (strict)"("Visible"=FALSE) -> ()  [unwired: 2 in, 2 out]
              }
              frame "Color Enable  **" {
                n199 = Index Array(array=w331, index=4) -> (element=w332:cluster{string[]})
                n200 = call <vilib>:"NT Read String.vi"("Name"=w334) -> ("String"=w333:string)  [unwired: 9 in, 1 out]
                n201 = Unbundle(w332) -> (w328:string[])
                n202 = Match First String(2:w328, 3:w333) -> (0:w329:i32)  [unwired: 1 out]
                n203 = property on="Test Ring" class="Ring (strict)"("Value"=w329, "Strings []"=w328) -> ()  [unwired: 2 in, 2 out]
                n204 = property on="Test Ring" class="Ring (strict)"("Visible"=TRUE) -> ()  [unwired: 2 in, 2 out]
                n205 = property on="Test Slider" class="Slide (strict)"("Visible"=FALSE) -> ()  [unwired: 2 in, 2 out]
              }
              frame Default {
                n206 = property on="Test Ring" class="Ring (strict)"("Visible"=FALSE) -> ()  [unwired: 2 in, 2 out]
                n207 = property on="Test Slider" class="Slide (strict)"("Visible"=FALSE) -> ()  [unwired: 2 in, 2 out]
              }
              frame "Brightness  **", "Color Level  **", "Compression  **", "FPS  **", "Sharpness  **" {
                n208 = call <vilib>:"NT Read Number.vi"("Name"=w340) -> ("Numeric"=w339:dbl)  [unwired: 9 in, 1 out]
                n209 = local write "Test Slider"(w339) -> ()
                n210 = property on="Test Slider" class="Slide (strict)"("Visible"=TRUE, "Scale.Maximum"=100.0 ("Scale.Range:Maximum")) -> ()  [unwired: 2 in, 2 out]
                n211 = property on="Test Ring" class="Ring (strict)"("Visible"=FALSE) -> ()  [unwired: 2 in, 2 out]
              }
            }
          }
        }
        n212 = property on="Progress" class="Clust (strict)"("Visible"=FALSE) -> ()  [unwired: 2 in, 2 out]
      }
      event "Test Name": Mouse Enter {
        # "Populate the ring with the list of tests"
        n213 = event-data() -> ()  [unwired: 1 in, 1 out]
        n214 = call <vilib>:"NT Read String Array.vi"("Name"="TestMode/TestList") -> ("String Array"=w348:string[])  [unwired: 9 in, 1 out]
        n215 = Build Array (concatenate)("Select the test to run...", w348) -> (w347:string[])
        n216 = property on="Test Name" class="Ring (strict)"("Strings []"=w347) -> ()  [unwired: 2 in, 2 out]
      }
      event "Test Name": Value Change {
        w350 = FALSE ("Visible")
        # "Tell the robot the test name to run"
        n217 = event-data() -> ("NewVal"=w354:u16)  [unwired: 1 in]
        n218 = property on="Test Name" class="Ring (strict)"() -> ("Strings []"=w355:string[])  [unwired: 2 in, 2 out]
        n219 = local write "Progress"(T6 {"Test Progress"=0, "Test Progress Text"=""} ("Progress")) -> ()
        n220 = Index Array(array=w355, index=w354) -> (element=w353:string)
        n221 = call <vilib>:"NT Write String.vi"("String"=w353, "Name"="TestMode/TestName") -> ()  [unwired: 9 in, 1 out]
        n222 = property on="Progress" class="Clust (strict)"("Visible"=TRUE) -> ()  [unwired: 2 in, 2 out]
        n223 = property on="Motor" class="Clust (strict)"("Visible"=w350) -> ()  [unwired: 2 in, 2 out]
        n224 = property on="Test Slider" class="Slide (strict)"("Visible"=w350) -> ()  [unwired: 2 in, 2 out]
        n225 = property on="On/Off" class="Bool (strict)"("Visible"=w350) -> ()  [unwired: 2 in, 2 out]
        n226 = property on="Rev/Fwd" class="Clust (strict)"("Visible"=w350) -> ()  [unwired: 2 in, 2 out]
        n227 = property on="Test Ring" class="Ring (strict)"("Visible"=w350) -> ()  [unwired: 2 in, 2 out]
      }
      event "Command Selection": Value Change {
        # "Get the params and show in table"
        n228 = event-data() -> ("NewVal"=w360:i32)  [unwired: 1 in]
        n229 = property on="Command Selection" class="MCListbox (strict)"() -> ("ItemNames"=w358:string[][])  [unwired: 2 in, 2 out]
        n230 = call <vilib>:"WPI_DashboardUpdate Command Params.vi"("NewVal"=w360, "Commands"=w358, "Param Tbl"=w359) -> ()  [unwired: 8 in, 1 out]
      }
      event "Execute Command": Value Change {
        # "Started one, Unique ID holds\nresponse"
        n231 = event-data() -> ()  [unwired: 1 in, 1 out]
        n232 = property on="Command Selection" class="MCListbox (strict)"() -> ("ItemNames"=w371:string[][])  [unwired: 2 in, 2 out]
        n233 = Index Array(array=w371, index (row)="Command Selection", index (col)=0) -> (element=w369:string)
        n234 = call <vilib>:"Invoke Commands.vi"("Command Params"="Command Params", "Function Name"=w369) -> ("Params"=w365:u8, "Started"=w364:bool)  [unwired: 7 in, 1 out]
        n235 = Array Subset(array="Command Params", length (row)=w365) -> (w366:string[][])  [unwired: 3 in]
        n236 = Select(t="Executing" ("Cmd Status"), s=w364, f="" ("Cmd Status")) -> (s? t:f=→"Cmd Status":string)
      }
      event "Command Selection": Double Click {
        n237 = event-data() -> ("Row"=w379:i32)  [unwired: 1 in]
        n238 = property on="Command Selection" class="MCListbox (strict)"() -> ("ItemNames"=w382:string[][])  [unwired: 2 in, 2 out]
        n239 = local read "Command Params"() -> (w378:string[][])
        n240 = Index Array(array=w382, index (row)=w379, index (col)=0) -> (element=w380:string)
        n241 = call <vilib>:"Invoke Commands.vi"("Command Params"=w378, "Function Name"=w380) -> ("Params"=w377:u8, "Started"=w372:bool)  [unwired: 7 in, 1 out]
        n242 = Array Subset(array=w378, length (row)=w377) -> (w376:string[][])  [unwired: 3 in]
        n243 = Select(t="Executing" ("Cmd Status"), s=w372, f="" ("Cmd Status")) -> (s? t:f=w373:string)
        n244 = local write "Cmd Status"(w373) -> ()
      }
      event "CheckList": Double Click {
        # "Shift clears all"
        # "Update symbols on the listbox"
        n245 = event-data() -> ("PlatMods.Shift"=w384:bool, "Row"=w386:i32)  [unwired: 1 in]
        n246 = case shown="True" w384 {
          tunnel: w386 -> [w390 _]
          tunnel: 1 -> [w389 _]
          frame False {
            n247 = property on="CheckList" class="LstBox (strict)"() -> ("Item Symbols"=w388:i32[])  [unwired: 2 in, 2 out]
            n248 = Replace Array Subset(array=w388, new element=w389, index=w390) -> (w387:i32[])
            n249 = property on="CheckList" class="LstBox (strict)"("Item Symbols"=w387) -> ()  [unwired: 2 in, 2 out]
          }
          frame True {
            w391 = 0 ("Top Row")
            n250 = property on="CheckList" class="LstBox (strict)"() -> ("Number of Rows"=w393:u32)  [unwired: 2 in, 2 out]
            n251 = Initialize Array(0, w393) -> (w392:i32[])
            n252 = property on="CheckList" class="LstBox (strict)"("Top Row"=w391, "Value"=w391, "Item Symbols"=w392) -> ()  [unwired: 2 in, 2 out]
          }
        }
      }
      event "CheckList": Key Down {
        # "Update symbols on the listbox\nLeft and right keys check and uncheck"
        n253 = event-data() -> ("VKey"=w397:T21)  [unwired: 1 in]
        n254 = case shown="\"Left\", \"Right\"" w397 {
          selector: w397 -> [w402 _]
          tunnel: eventvkey."Left" ("VKey") -> [w400 _]
          frame "Left", "Right" {
            n255 = Equal?(x=w400, y=w402) -> (x = y?=w401:bool)
            n256 = Select(t=0, s=w401, f=1) -> (s? t:f=w403:i32)
            n257 = property on="CheckList" class="LstBox (strict)"() -> ("Item Symbols"=w406:i32[])  [unwired: 2 in, 2 out]
            n258 = Replace Array Subset(array=w406, new element=w403, index="CheckList") -> (w405:i32[])
            n259 = property on="CheckList" class="LstBox (strict)"("Item Symbols"=w405) -> ()  [unwired: 2 in, 2 out]
          }
          frame Default {
          }
        }
      }
      event "Motor.Enable": Value Change {
        # "When the test mode otor enable helper is set, update that\ntree row item's value"
        n260 = event-data() -> ("NewVal"=w412:bool)  [unwired: 1 in]
        n261 = Unbundle("Motor") -> ("Value"=w411:dbl)  [unwired: 1 out]
        n262 = Select(t=w411, s=w412, f=0.0) -> (s? t:f=w409:dbl)
        n263 = call <vilib>:"NT Write Number.vi"("Numeric"=w409, "Name"=w408) -> ()  [unwired: 9 in, 1 out]
      }
      event "Test Slider": Value Change {
        # "When the test mode slider helper is set, update that\ntree row item's value"
        n264 = event-data() -> ("NewVal"=w415:dbl)  [unwired: 1 in]
        n265 = call <vilib>:"NT Write Number.vi"("Numeric"=w415, "Name"=w416) -> ()  [unwired: 9 in, 1 out]
      }
      event "On/Off": Value Change {
        # "When the test mode on/off helper value is set, update that\ntree row item's value"
        n266 = event-data() -> ("NewVal"=w420:bool)  [unwired: 1 in]
        n267 = Boolean To (0,1)(Boolean=w420) -> (0, 1=w419:i16)
        n268 = call <vilib>:"NT Write Number.vi"("Numeric"=w419, "Name"=w418) -> ()  [unwired: 9 in, 1 out]
      }
      event "Rev/Fwd": Value Change {
        # "When the test mode helper value for relays is set, update that\ntree row item's value"
        n269 = event-data() -> ("NewVal.Forward"=w428:bool, "NewVal.Reverse"=w427:bool)  [unwired: 1 in]
        n270 = Boolean To (0,1)(Boolean=w428) -> (0, 1=w424:i16)
        n271 = Boolean To (0,1)(Boolean=w427) -> (0, 1=w426:i16)
        n272 = Negate(x=w426) -> (-x=w425:i16)
        n273 = Add(x=w424, y=w425) -> (x+y=w423:i16)
        n274 = call <vilib>:"NT Write Number.vi"("Numeric"=w423, "Name"=w422) -> ()  [unwired: 9 in, 1 out]
      }
      event "Test Ring": Value Change {
        # "When a test mode helper value is selected from the ring,\nset the tree item's variable to the string value"
        n275 = event-data() -> ("NewVal"=w432:u16)  [unwired: 1 in]
        n276 = property on="Test Ring" class="Ring (strict)"() -> ("Strings []"=w433:string[])  [unwired: 2 in, 2 out]
        n277 = Index Array(array=w433, index=w432) -> (element=w431:string)
        n278 = call <vilib>:"NT Write String.vi"("String"=w431, "Name"=w430) -> ()  [unwired: 9 in, 1 out]
      }
      event "Rec Mode": Value Change {
        # "Update globals for recording mode and path to read log from.\nClear when logging and let NetworkTables set path for vision to\nuse."
        n279 = event-data() -> ("NewVal"=w444:enum32{"Stop", "Record", "Playback"})  [unwired: 1 in]
        n280 = global write "WPI_DashboardLogging Global.vi" "Logging Filename"(path "") -> ()
        n281 = global write "WPI_DashboardLogging Global.vi" "Recording"(w444) -> ()
        n282 = case shown="\"Playback\"" w444 {
          tunnel: w443 -> [_ w446 w455]
          tunnel: [_ _ w454] -> w441
          tunnel: [_ _ w453] -> _
          tunnel: w439 -> [_ _ w451]
          tunnel: cluster{i32, i32} {-250, 170} -> [_ _ w450]
          tunnel: [_ _ T22 {"Image Size"=TRUE, "Image Type"=TRUE, "Pixel Value"=TRUE, "ROI Information"=TRUE, "Zoom Factor"=FALSE} ("Image Information Shown:All Elements")] -> w434
          tunnel: [_ _ TRUE ("Zoom Factor")] -> w435
          tunnel: w437 -> [_ _ w447]
          frame Default {
          }
          frame "Stop", "Record" {
            # "Place Window too"
            n283 = invoke class="VI" method="FP.Close"(reference=w446) -> (reference out=w445:refnum<vi>)  [unwired: 2 in, 2 out]
            n284 = invoke class="VI" method="Abort VI"(reference=w445) -> ()  [unwired: 2 in, 3 out]
          }
          frame "Playback" {
            n285 = call "Open Playback Panel.vi"("Offset"=w450, "DB VI Ref"=w451, "Playback in"=w455) -> ("Playback out"=w452:refnum<vi>)  [unwired: 8 in]
            n286 = register-events(w452, w447) -> (reference out=w454:refnum<event-registration>, error out=w453:errorcluster)  [unwired: 2 in]
          }
        }
        n287 = property on="Camera Image Right" class="ImageControl"("Image Information Shown"=w434, "Image Information Visible"=w435) -> ()  [unwired: 2 in, 2 out]
        n288 = property on="Camera Image" class="ImageControl"("Image Information Shown"=w434, "Image Information Visible"=w435) -> ()  [unwired: 2 in, 2 out]
        n289 = call <vilib>:"WPI_DashboardNT Log FieldName Cache.vi"("Operation"=enum16{"Lookup/Add", "Index", "Clear"}."Clear") -> ()  [unwired: 8 in, 3 out]
      }
      event Panel Close {
        w457 = enum32{"Stop", "Record", "Playback"}."Stop" ("Rec Mode")
        # "Playback window has been closed, abort"
        n290 = event-data() -> ()  [unwired: 1 in, 4 out]
        n291 = local write "Rec Mode"(w457) -> ()
        n292 = global write "WPI_DashboardLogging Global.vi" "Recording"(w457) -> ()
      }
      event Panel Close {
        # "Abort playback window and ourself"
        n293 = event-data() -> ()  [unwired: 1 in, 4 out]
        n294 = invoke class="VI" method="FP.Close"(reference=w461) -> (reference out=w460:refnum<vi>)  [unwired: 2 in, 2 out]
        n295 = invoke class="VI" method="Abort VI"(reference=w460) -> (error out=w459:errorcluster)  [unwired: 2 in, 2 out]
        n296 = invoke class="VI" method="Abort VI"(error in=w459) -> ()  [unwired: 2 in, 3 out]
      }
      event User Event {
        n297 = event-data() -> ("IDs"=w468:cluster{"RPC field ID":u16, "Unique ID":u16}, "String"=w467:string)  [unwired: 1 in]
        n298 = Bundle("IDs"=w468, "String"=w467) -> (w466:T9)  [unwired: 1 in]
        n299 = call <vilib>:"Retrieve RPC Response.vi"("RPC Response"=w466) -> ("Output"=w464:string[][])  [unwired: 10 in]
        n300 = Build Array (concatenate)(w462, w464) -> (w463:string[][])
        n301 = local write "Command Params"(w463) -> ()
        n302 = local write "Cmd Status"("" ("Cmd Status")) -> ()
      }
      event "Tree": Double Click {
        n303 = event-data() -> ("PlatMods"=w474:T25, "Tag"=w471:string)  [unwired: 1 in]
        n304 = Unbundle(w474) -> ("Shift"=w473:bool)  [unwired: 4 out]
        n305 = String Subset(string=w471, length (rest)=1 ("length (rest)")) -> (substring=w470:string)  [unwired: 1 in]
        n306 = Not(x=w473) -> (.not. x?=w472:bool)
        n307 = case shown="\"/\"" w470 {
          tunnel: w471 -> [_ w477]
          tunnel: w472 -> [_ w476]
          frame Default {
          }
          frame "/" {
            n308 = call <vilib>:"NT Update Persistence.vi"("Persistence"=w476, "Name"=w477) -> ()  [unwired: 9 in, 1 out]
          }
        }
      }
    }
  }
  n309 = while {
    tunnel: w63 -> [w479]
    i -> [w482]
    stop <- FALSE stop-if-true
    n310 = Wait (ms)(milliseconds to wait=u32 100) -> ()  [unwired: 1 out]
    n311 = case shown="\"Playback\"" "Rec Mode" {
      tunnel: w482 -> [_ _ w497]
      tunnel: [u32 2829099 ("Base Color") u32 11141120 ("Target Color") w486] -> w478
      frame "Stop", Default {
        # "Reset the color, extra updates don't cost much"
      }
      frame "Record" {
      }
      frame "Playback" {
        # "Playback"
        n312 = Quotient & Remainder(x=w497, y=u32 50 ("milliseconds to wait")) -> (x-y*floor(x/y)=w493:u32)  [unwired: 1 out]
        n313 = Divide(x=w493, y=u32 50 ("milliseconds to wait")) -> (x/y=w490:dbl)
        n314 = Multiply(x=6.283185307179586, y=w490) -> (x*y=w495:dbl)
        n315 = Sine(x=w495) -> (sin(x)=w494:dbl)
        n316 = Absolute Value(x=w494) -> (abs(x)=w487:dbl)
        n317 = call "Interpolate RGB Color.vi"("Proportion"=w487, "Target Color"=u32 30976, "Base Color"=u32 2829099) -> ("Result Color"=w486:u32)  [unwired: 8 in]
      }
    }
    n318 = property class="Pane"(reference=w479, "PaneColor"=w478) -> ()  [unwired: 1 in, 2 out]
  }
  n319 = local write "Dashboard Tab"(T2."Drive" ("Dashboard Tab")) -> ()
  n320 = property on="On/Off" class="Bool (strict)"("Visible"=w34) -> ()  [unwired: 2 in, 2 out]
  n321 = property on="Motor" class="Clust (strict)"("Visible"=w34) -> ()  [unwired: 2 in, 2 out]
  n322 = property on="Progress" class="Clust (strict)"("Visible"=w34) -> ()  [unwired: 2 in, 2 out]
  n323 = property on="Test Ring" class="Ring (strict)"("Visible"=w34) -> ()  [unwired: 2 in, 2 out]
  n324 = property on="Rev/Fwd" class="Clust (strict)"("Visible"=w34) -> ()  [unwired: 2 in, 2 out]
  n325 = while {
    tunnel: u16 1741 ("timeout ms (25000)") -> [w499]
    stop <- FALSE stop-if-true
    n326 = TCP Create Listener(10:w499) -> (0:w498:errorcluster, 3:w500:refnum<k5>)  [unwired: 4 in, 1 out]
    n327 = case shown="No Error" w498 {
      selector: w498 -> [w502 _]
      tunnel: w500 -> [w503 _]
      frame No Error {
        n328 = while {
          tunnel: w503 -> [w506]
          tunnel: w502 -> [w505]
          stop <- FALSE stop-if-true
          n329 = TCP Wait On Listener(8:w505, 11:w506) -> (0:w507:errorcluster, 4:w508:refnum<k5>)  [unwired: 2 in, 3 out]
          n330 = local write "TCP"(w508) -> ()
          n331 = case shown="No Error" w507 {
            frame No Error {
            }
            frame Error {
              n332 = Wait (ms)(milliseconds to wait=u32 1000) -> ()  [unwired: 1 out]
            }
          }
        }
      }
      frame Error {
        n333 = Wait (ms)(milliseconds to wait=u32 1000) -> ()  [unwired: 1 out]
      }
    }
  }
  n334 = local write "Command Selection"(u16 0 ("milliseconds to wait")) -> ()
  n335 = local write "Command Params"(string[][] [] ("Command Params")) -> ()
  n336 = global write "WPI_DashboardLogging Global.vi" "Recording"(w57) -> ()
  n337 = local write "Rec Mode"(w57) -> ()
